vi "ConfigExportPosList.vi"(0 "XML File Path":path, 1 "Array":string[][](array[string]), 3 "error in (no error)":errorcluster, 4 "Only Pos":bool) -> (7 "XML File Path Out":path, 10 "error out":errorcluster)   [LabVIEW 2018]
uses:
  <vilib>/Utility/xml.llb/Write to XML File(array).vi
  <vilib>/Utility/xml.llb/Read From XML File(array).vi
panel:
  out "XML Elements":string[](array[string])
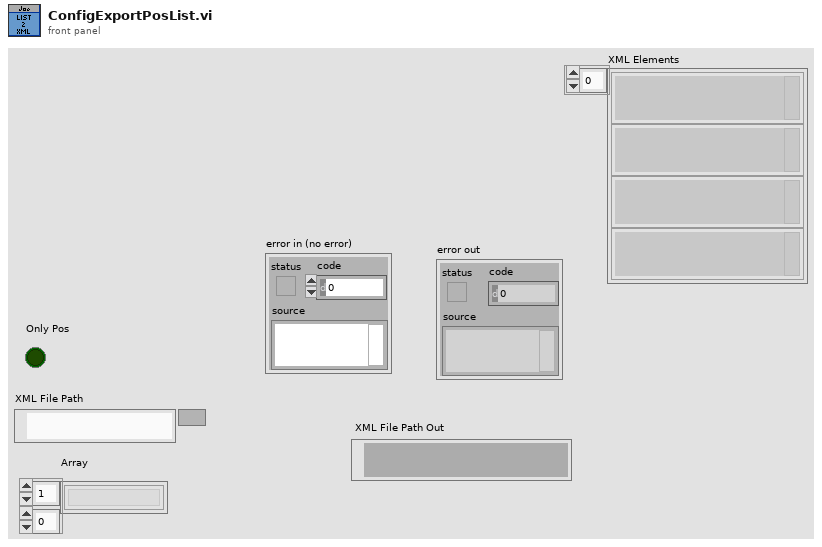
[diagram p1: front panel]
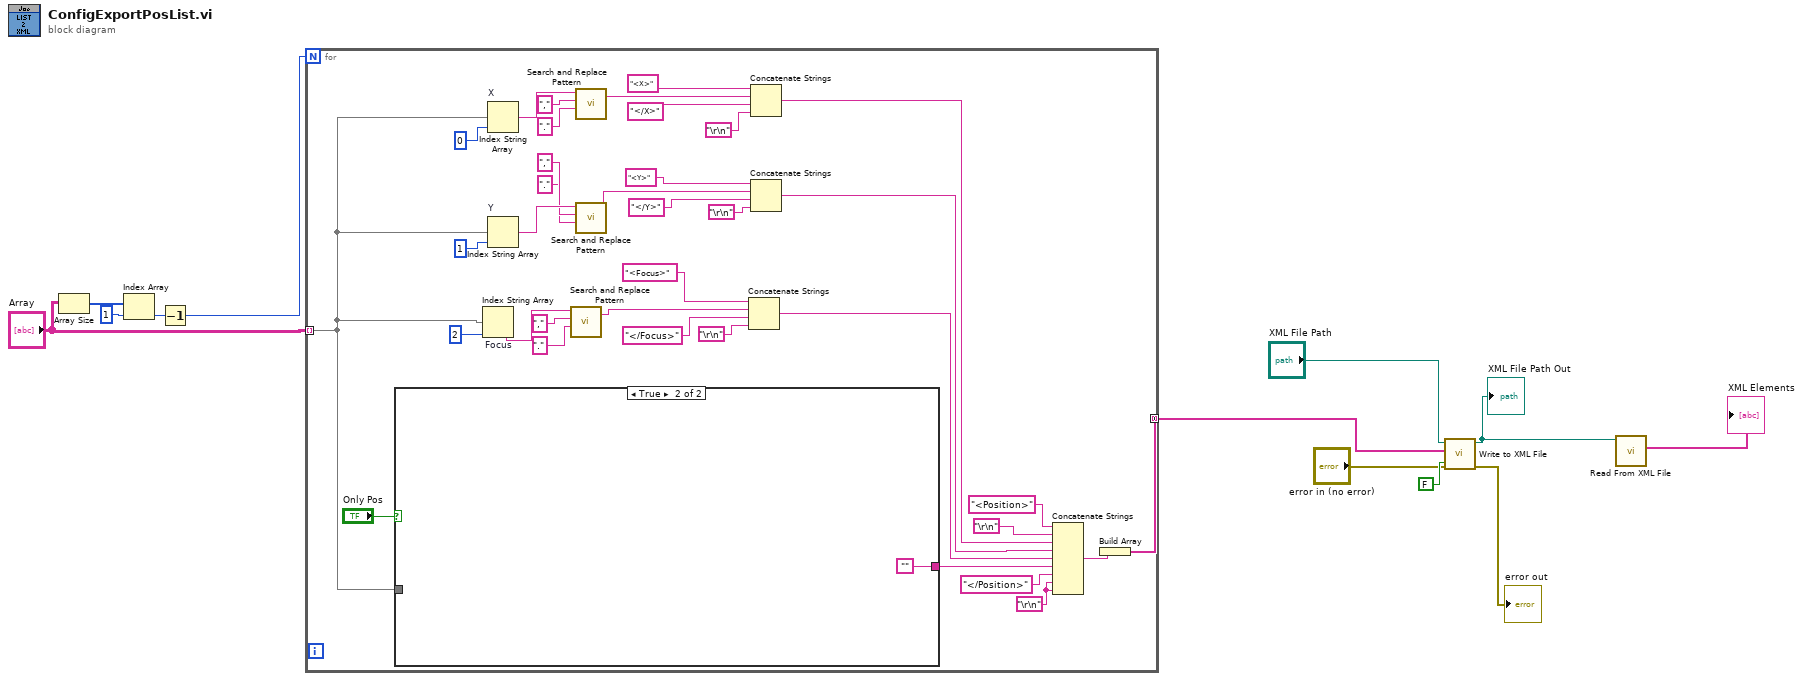
[diagram p0: block diagram]
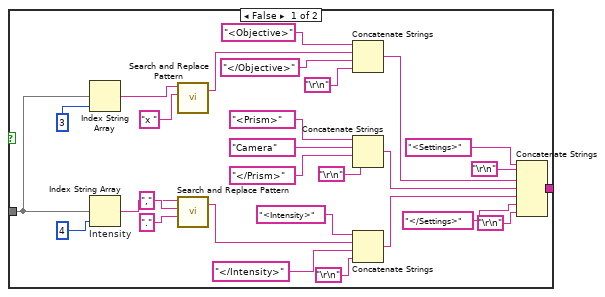
[diagram p2: hidden frame]
diagram:
  n1 = Array Size(array="Array") -> (size(s)=w6:i32[])
  n2 = Index Array(array=w6, index=1) -> (element=w4:i32)
  n3 = Decrement(x=w4) -> (x-1=w9:i32)
  n4 = for {
    N: w9 -> [_]
    tunnel: "Array" -> [w15] mode=indexing
    tunnel: [w39] -> w12 mode=concatenating
    w32 = "\r\n"
    n5 = case shown="True" "Only Pos" {
      tunnel: [w72 ""] -> w43
      tunnel: w15 -> [w49 _]
      frame False {
        n6 = Index String Array(1:3 ("index"), 2:w49) -> (0:w56:string)  [unwired: 1 in]
        n7 = Index String Array "Intensity"(1:4 ("index"), 2:w49) -> (0:w51:string)  [unwired: 1 in]
        n8 = call <vilib>:"Search and Replace Pattern.vi"("string"=w56, "regular expression (\"\")"="x " ("replace string (\"\")")) -> ("result string"=w54:string)  [unwired: 3 in, 1 out]
        n9 = call <vilib>:"Search and Replace Pattern.vi"("string"=w51, "regular expression (\"\")"="," ("regular expression (\"\")"), "replace string (\"\")"="." ("replace string (\"\")")) -> ("result string"=w50:string)  [unwired: 2 in, 1 out]
        n10 = Concatenate Strings("<Objective>" ("string"), w54, "</Objective>" ("string"), "\r\n") -> (w66:string)
        n11 = Concatenate Strings("<Prism>" ("output string"), "Camera" ("output string"), "</Prism>" ("output string"), "\r\n") -> (w61:string)
        n12 = Concatenate Strings("<Intensity>" ("output string"), w50, "</Intensity>", "\r\n") -> (w57:string)
        n13 = Concatenate Strings("<Settings>" ("string"), "\r\n", w66, w61, w57, "</Settings>" ("string"), "\r\n") -> (w72:string)
      }
      frame True {
      }
    }
    n14 = Index String Array "Focus"(1:2 ("index"), 2:w15) -> (0:w22:string)  [unwired: 1 in]
    n15 = Index String Array "X"(1:0 ("index"), 2:w15) -> (0:w25:string)  [unwired: 1 in]
    n16 = Index String Array "Y"(1:1 ("index"), 2:w15) -> (0:w31:string)  [unwired: 1 in]
    n17 = call <vilib>:"Search and Replace Pattern.vi"("string"=w22, "regular expression (\"\")"="," ("regular expression (\"\")"), "replace string (\"\")"="." ("replace string (\"\")")) -> ("result string"=w23:string)  [unwired: 2 in, 1 out]
    n18 = call <vilib>:"Search and Replace Pattern.vi"("string"=w25, "regular expression (\"\")"="," ("regular expression (\"\")"), "replace string (\"\")"="." ("replace string (\"\")")) -> ("result string"=w24:string)  [unwired: 2 in, 1 out]
    n19 = call <vilib>:"Search and Replace Pattern.vi"("string"=w31, "regular expression (\"\")"="," ("regular expression (\"\")"), "replace string (\"\")"="." ("replace string (\"\")")) -> ("result string"=w28:string)  [unwired: 2 in, 1 out]
    n20 = Concatenate Strings("<Focus>" ("string"), w23, "</Focus>" ("string"), "\r\n") -> (w14:string)
    n21 = Concatenate Strings("<X>" ("string"), w24, "</X>" ("string"), "\r\n") -> (w42:string)
    n22 = Concatenate Strings("<Y>" ("string"), w28, "</Y>" ("string"), "\r\n") -> (w41:string)
    n23 = Concatenate Strings("<Position>" ("string"), "\r\n", w42, w41, w14, w43, "</Position>" ("string"), w32, w32) -> (w40:string)
    n24 = Build Array(w40) -> (w39:string[])
  }
  n25 = call-poly <vilib>:"Write to XML File.vi"("Standalone? (T)"=FALSE, "error in (no error)"="error in (no error)", "XML Input"=w12, "XML File Path"="XML File Path") -> ("error out"=→"error out":errorcluster, "XML File Path"=w3:path)  [unwired: 5 in, 1 out]
  "XML File Path Out" <- w3
  n26 = call-poly <vilib>:"Read From XML File.vi"("XML File Path"=w3) -> ("XML Elements"=→"XML Elements":string[])  [unwired: 8 in, 2 out]
